vi "3 - Use a DAQmx Task (Solution).vi"() -> ()   [LabVIEW 2012]
uses:
  <vilib>/DAQmx/read.llb/DAQmx Read (Analog 1D Wfm NChan NSamp).vi
  <vilib>/DAQmx/miscellaneous.llb/DAQmx Fill In Error Info.vi
panel:
  out "Alarm Output":bool
  in  "Alarm Level":dbl=26.0
  out "Temperature":waveform(dbl)[](graph)
  in  "stop":bool
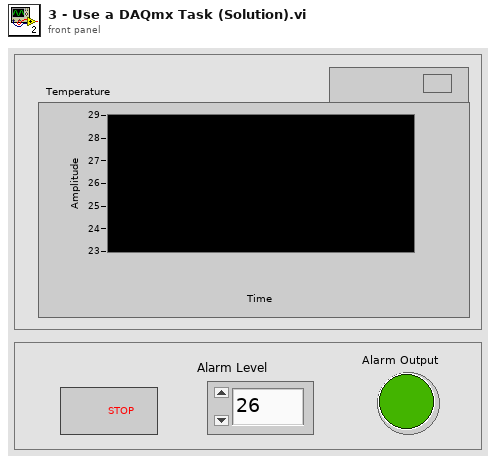
[diagram p1: front panel]
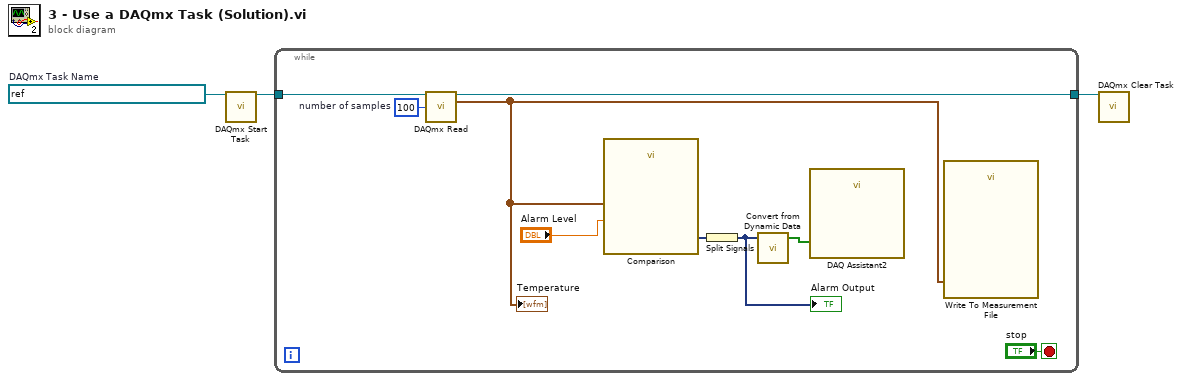
[diagram p0: block diagram]
diagram:
  w1 = refnum<k21> "Measure Temperature and Light"  # DAQmx Task Name
  n1 = call <vilib>:"DAQmx Start Task.vi"("task/channels in"=w1) -> ("task out"=w3:refnum<k21>)  [unwired: 13 in, 1 out]
  n2 = while {
    tunnel: w3 -> [w8]
    tunnel: [w7] -> w2
    stop <- "stop" stop-if-true
    w5 = 100  # number of samples
    n3 = call-poly <vilib>:"DAQmx Read.vi"("task/channels in"=w8, "number of samples per channel"=w5) -> ("task out"=w7:refnum<k21>, "data"=w6:waveform(dbl)[])  [unwired: 11 in, 1 out]
    "Temperature" <- w6
    n4 = call "Comparison"("Operand 2"="Alarm Level", "Operand 1"=w6) -> ("Result"=w10:dynamicdata)  [unwired: 1 in, 8 out]
    n5 = Split Signals(w10) -> (w4:dynamicdata)  [unwired: 1 in]
    "Alarm Output" <- w4
    n6 = call "Convert from Dynamic Data"("Dynamic Data Type"=w4) -> ("Array"=w9:bool[])  [unwired: 3 in]
    n7 = call "DAQ Assistant2"("data"=w9) -> ()  [unwired: 4 in, 15 out]
    n8 = call "Write To Measurement File"("Signals"=w6) -> ()  [unwired: 16 in, 3 out]
  }
  n9 = call <vilib>:"DAQmx Clear Task.vi"("task in"=w2) -> ()  [unwired: 14 in, 1 out]
